vi "testUintInRangeCoerce.vi"(8 "error in (no error)":errorcluster, 11 "TestCase in":refnum<class "UnitTestUintClass.lvclass">) -> (0 "error out":errorcluster, 3 "TestCase out":refnum<class "UnitTestUintClass.lvclass">)   [LabVIEW 2011, in "UnitTestUintClass.lvclass"]
uses:
  UnitTestUintClass.lvclass
  UnitTestUintClass.lvclass/UnitTestUintClass.ctl
  UintClass/uintInRangeCoerceELowerEUpper.vi
  <vilib>/addons/_JKI Toolkits/VI Tester/TestCase.llb/TestCase.lvclass
  UintClass/UintClass.lvclass
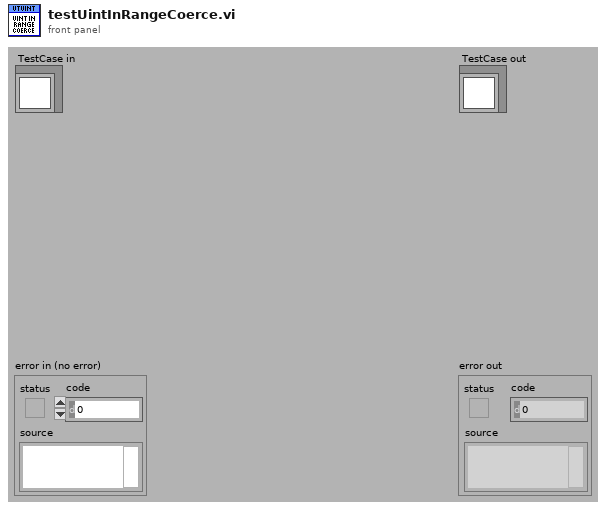
[diagram p1: front panel]
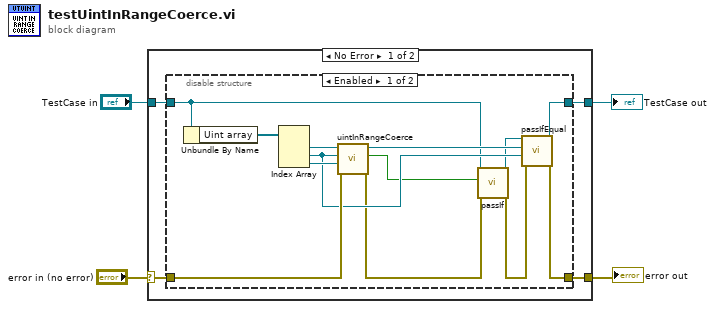
[diagram p0: block diagram]
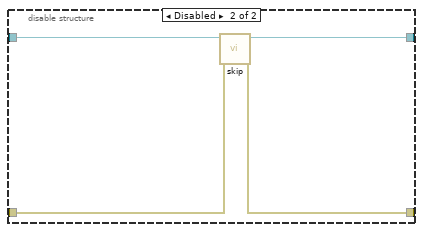
[diagram p2: hidden frame]
diagram:
  n1 = case shown="No Error" "error in (no error)" {
    selector: "error in (no error)" -> [w6 w27]
    tunnel: [w5 w27] -> w3
    tunnel: [w7 w26] -> w1
    tunnel: "TestCase in" -> [w8 w26]
    frame No Error {
      n2 = disable-structure shown="Enabled" {
        disable-tunnel: w8 -> [w12 w25]
        disable-tunnel: [w21 w22] -> w7
        disable-tunnel: w6 -> [w16 w24]
        disable-tunnel: [w20 w23] -> w5
        frame Enabled {
          n3 = Unbundle By Name(w12) -> ("Uint array"=w19:refnum<class "UintClass.lvclass">[])
          n4 = Index Array(array=w19) -> (element #1=w18:refnum<class "UintClass.lvclass">, element #2=w14:refnum<class "UintClass.lvclass">, element #3=w17:refnum<class "UintClass.lvclass">)  [unwired: 3 in]
          n5 = call-poly "uintInRangeCoerce.vi"("Error in (no error)"=w16, "Lowerlimit"=w17, "Int in"=w14, "Upperlimit"=w18) -> ("Error out"=w10:errorcluster, "In Range?"=w13:bool, "Coerced(Int)"=w15:refnum<class "UintClass.lvclass">)  [unwired: 4 in, 1 out]
          n6 = call-dynamic "passIf.vi"("error in (no error)"=w10, "pass"=w13, "TestCase in"=w12) -> ("error out"=w9:errorcluster, "TestCase out"=w11:refnum<class "UnitTestUintClass.lvclass">)  [unwired: 7 in]
          n7 = call-dynamic "passIfEqual.vi"("error in (no error)"=w9, "y"=w14, "x"=w15, "TestCase in"=w11) -> ("error out"=w20:errorcluster, "TestCase out"=w21:refnum<class "UnitTestUintClass.lvclass">)  [unwired: 6 in]
        }
        frame Disabled {
          n8 = call <vilib>:"skip.vi"("error in (no error)"=w24, "TestCase in"=w25) -> ("error out"=w23:errorcluster, "TestCase out"=w22:refnum<class "UnitTestUintClass.lvclass">)  [unwired: 8 in]
        }
      }
    }
    frame Error {
    }
  }
  "error out" <- w3
  "TestCase out" <- w1
